vi "Oil Pump Control.vi"(0 "Session Handle in":T1, 5 "On?":bool, 11 "error in (no error)":errorcluster) -> (4 "Session Handle out":T1, 6 "Failure Reason":string, 8 "Success?":bool, 15 "error out":errorcluster)   [LabVIEW 2015, in "Oil.lvclass"]
uses:
  Oil.lvclass
  Typedefs/Session Handle.ctl
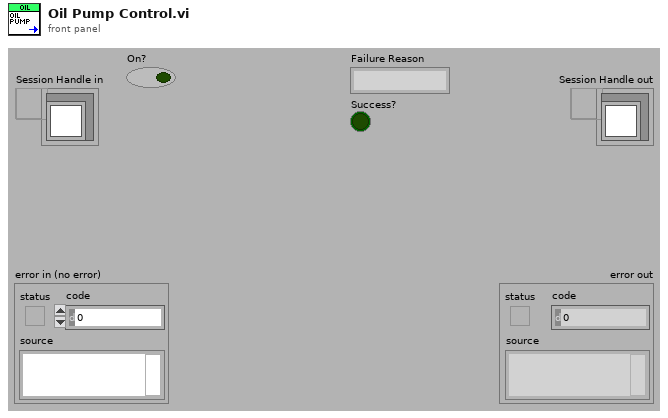
[diagram p1: front panel]
types:
  T1 = typedef "Oil.lvclass/Session Handle.ctl" = refnum<data-value>
  T2 = typedef "XNET Frame CAN.ctl" = cluster{"timestamp":timestamp, "payload":u8[], "identifier":u32, "type":T3, "extended?":bool, "echo?":bool}
  T3 = typedef "XNET Frame Type CAN.ctl" = u8
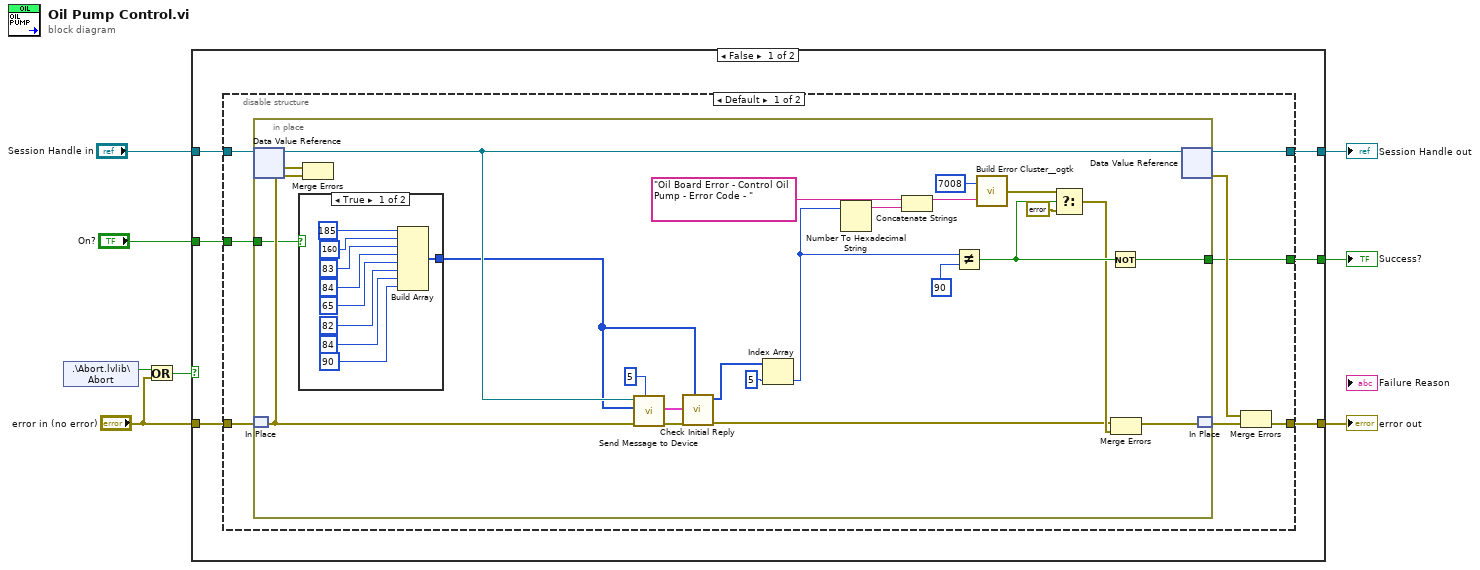
[diagram p0: block diagram]
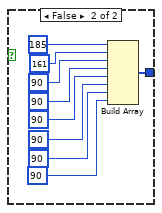
[diagram p2: hidden frame]
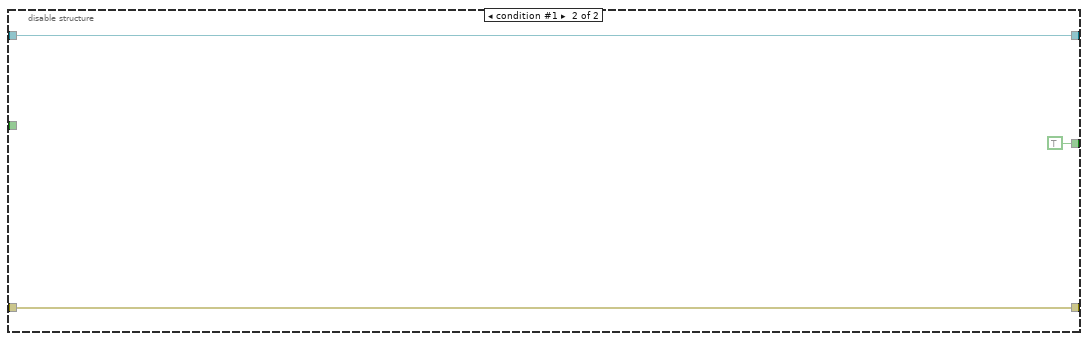
[diagram p3: hidden frame]
diagram:
  n1 = shared-variable ".\\Abort.lvlib\\Abort"() -> (w4:bool)  [unwired: 1 in, 1 out]
  n2 = Or(x=w4, y="error in (no error)") -> (x .or. y?=w3:bool)
  n3 = case shown="False" w3 {
    tunnel: "Session Handle in" -> [w14 w68]
    tunnel: [w13 w68] -> w7
    tunnel: [w12 w67] -> w6
    tunnel: "On?" -> [w11 _]
    tunnel: "error in (no error)" -> [w10 w67]
    tunnel: [w9 _] -> w1
    frame False {
      n4 = disable-structure shown="Default" {
        disable-tunnel: w14 -> [w22 w66]
        disable-tunnel: [w21 w66] -> w13
        disable-tunnel: [w18 w64] -> w12
        disable-tunnel: w11 -> [w17 _]
        disable-tunnel: w10 -> [w16 w64]
        disable-tunnel: [w15 TRUE] -> w9
        frame condition #0 (active) {
          n5 = in-place {
            in-place-border: w17 -> [w39]
            in-place-border: [w27] -> w15
            n6 = in-place-dvr #1(w22) -> (w41:refnum<class "Oil.lvclass">, w45:errorcluster)
            n7 = in-place-match #2(w16) -> (w42:errorcluster)
            n8 = case shown="True" w39 {
              tunnel: [w46 w55] -> w38
              frame True {
                n9 = Build Array(u8 185 ("new element/subarray"), u8 160 ("new element/subarray"), u8 83 ("new element/subarray"), u8 84 ("new element/subarray"), u8 65 ("new element/subarray"), u8 82 ("new element/subarray"), u8 84 ("new element/subarray"), u8 90 ("new element/subarray")) -> (w46:u8[])
              }
              frame False {
                n10 = Build Array(u8 185 ("new element/subarray"), u8 161 ("new element/subarray"), u8 90 ("new element/subarray"), u8 90 ("new element/subarray"), u8 90 ("new element/subarray"), u8 90 ("new element/subarray"), u8 90 ("new element/subarray"), u8 90 ("new element/subarray")) -> (w55:u8[])
              }
            }
            n11 = Merge Errors(w42, w45) -> ()  [unwired: 1 out]
            n12 = call "Send Message to Device.vi"("Number of Retries"=5, "error in (no error)"=w42, "payload"=w38, "CAN Comm In"=w41) -> ("error out"=w24:errorcluster, "Reply"=w43:T2[])  [unwired: 5 in, 1 out]
            n13 = call "Check Initial Reply.vi"("Write Message"=w38, "error in (no error)"=w24, "Reply"=w43) -> ("error out"=w23:errorcluster, "Data Packet 2"=w40:u8[])  [unwired: 5 in, 2 out]
            n14 = Index Array(array=w40, index=5) -> (element=w28:u8)
            n15 = Number To Hexadecimal String(2:w28) -> (0:w30:string)  [unwired: 1 in]
            n16 = Concatenate Strings("Oil Board Error - Control Oil Pump - Error Code - " ("string"), w30) -> (w35:string)
            n17 = Not Equal?(x=w28, y=u8 90 ("new element/subarray")) -> (x != y?=w31:bool)
            n18 = call <userlib>:"Build Error Cluster__ogtk.vi"("String to Prepend to source (\"\")"=w35, "code"=7008) -> ("error out"=w33:errorcluster)
            n19 = Select(t=w33, s=w31, f=errorcluster {"status"=FALSE, "code"=0, "source"=""}) -> (s? t:f=w26:errorcluster)
            n20 = Not(x=w31) -> (.not. x?=w27:bool)
            n21 = Merge Errors(w23, w26) -> (w25:errorcluster)
            n22 = in-place-dvr #1(w41) -> (w21:T1, w19:errorcluster)
            n23 = in-place-match #2(w25) -> (w20:errorcluster)
          }
          n24 = Merge Errors(w19, w20) -> (w18:errorcluster)
        }
        frame condition #1 {
        }
      }
    }
    frame True {
    }
  }
  "Session Handle out" <- w7
  "error out" <- w6
  "Success?" <- w1
